vi "Multiclamp Auto Pipette Offeset.vi"(8 "error in (no error)":errorcluster, 9 "pnError":i32, 11 "hMCCmsg":i32) -> (0 "error out":errorcluster, 1 "pnError out":i32, 3 "hMCCmsg":i32)   [LabVIEW 2012, in "MultiClamp 700B Controls.lvlib"]
uses:
  MultiClamp 700B Controls.lvlib
  AxMultiClampMsg/AxMultiClampMsg.lvlib
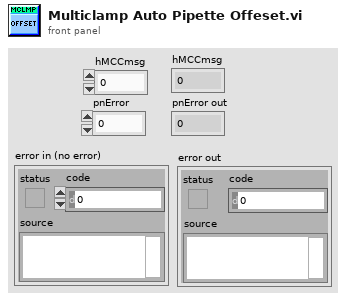
[diagram p1: front panel]
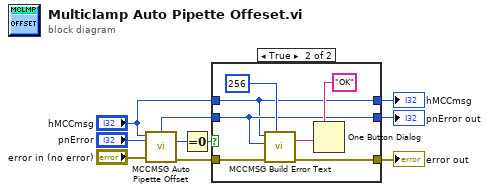
[diagram p0: block diagram]
diagram:
  n1 = call "MCCMSG Auto Pipette Offset.vi"("error in (no error)"="error in (no error)", "pnError"="pnError", "hMCCmsg"="hMCCmsg") -> ("error out"=w9:errorcluster, "pnError out"=w1:i32, "function return"=w8:i32)  [unwired: 6 in]
  n2 = Equal To 0?(x=w8) -> (x = 0?=w10:bool)
  n3 = case shown="True" w10 {
    tunnel: w1 -> [w13 w16]
    tunnel: w9 -> [w11 w20]
    tunnel: "hMCCmsg" -> [w12 w15]
    tunnel: [w13 w16] -> w4
    tunnel: [w12 w15] -> w5
    tunnel: [w11 w14] -> w3
    frame False {
    }
    frame True {
      n4 = call "MCCMSG Build Error Text.vi"("uMaxLen"=u32 256, "error in (no error)"=w20, "nErrorNum"=w16, "hMCCmsg"=w15) -> ("error out"=w14:errorcluster, "sTxtBuf out"=w19:string)  [unwired: 5 in, 1 out]
      n5 = One Button Dialog(message=w19, button name ("OK")="OK") -> ()  [unwired: 1 out]
    }
  }
  "hMCCmsg" <- w5
  "pnError out" <- w4
  "error out" <- w3
